vi "Add Sheets.vi"(8 "error in":errorcluster, 9 "Write/Read Cell":T1={"Cell Range"="", "Data 2D"=[], "Select Sheet"="", "1 Data"="", "Data 1D"=[], "Font col"=0, "Bold"=TRUE, "Font Size"=18, "Inside lines"=FALSE}, 10 "Work Sheet":refnum<k7>, 11 "Excel._Workbook":refnum<k7>) -> (0 "error out":errorcluster, 2 "Work Sheet":refnum<k7>, 3 "Excel._Workbook":refnum<k7>)   [LabVIEW 2017]
uses:
  controls/read.write.ctl
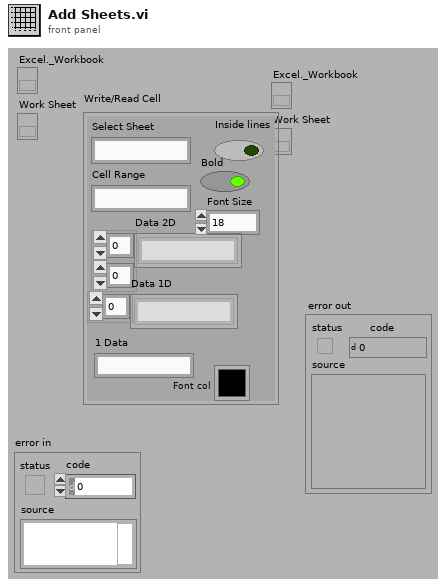
[diagram p1: front panel]
types:
  T1 = typedef "read.write.ctl" = cluster{"Cell Range":string, "Data 2D":string[][], "Select Sheet":string, "1 Data":string, "Data 1D":string[], "Font col":u32, "Bold":bool, "Font Size":i32, "Inside lines":bool}
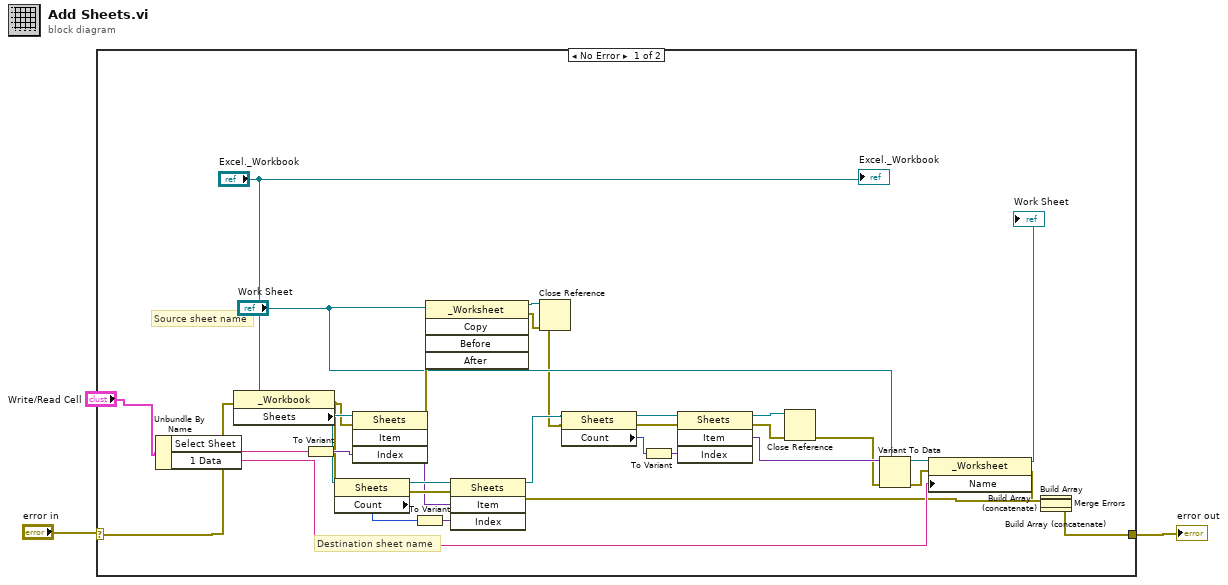
[diagram p0: block diagram]
diagram:
  n1 = case shown="No Error" "error in" {
    selector: "error in" -> [w30 w39]
    tunnel: [w7 w39] -> w1
    frame No Error {
      # "Source sheet name"
      # "Destination sheet name"
      n2 = Unbundle By Name("Write/Read Cell") -> ("Select Sheet"=w29:string, "1 Data"=w28:string)
      n3 = property class="_Workbook"(reference="Excel._Workbook", error in=w30) -> (error out=w15:errorcluster, "Sheets"=w16:refnum<k7>)  [unwired: 1 out]
      n4 = To Variant(anything=w29) -> (Variant=w32:variant)
      n5 = property class="Sheets"(reference=w16, error in=w15) -> (reference out=w17:refnum<k7>, error out=w18:errorcluster, "Count"=w13:i32)
      n6 = invoke class="Sheets" method="Item"(reference=w16, error in=w15, "Index"=w32) -> (error out=w25:errorcluster)  [unwired: 1 in, 3 out]
      n7 = To Variant(anything=w13) -> (Variant=w14:variant)
      n8 = invoke class="Sheets" method="Item"(reference=w17, error in=w18, "Index"=w14) -> (reference out=w11:refnum<k7>, error out=w9:errorcluster, "Item"=w12:variant)  [unwired: 1 in, 1 out]
      n9 = invoke class="_Worksheet" method="Copy"(reference="Work Sheet", error in=w25, "After"=w12) -> (reference out=w27:refnum<k7>, error out=w26:errorcluster)  [unwired: 2 in, 3 out]
      n10 = Close Reference(reference=w27, error in (no error)=w26) -> (error out=w10:errorcluster)
      n11 = property class="Sheets"(reference=w11, error in=w10) -> (reference out=w20:refnum<k7>, error out=w19:errorcluster, "Count"=w22:i32)
      n12 = To Variant(anything=w22) -> (Variant=w33:variant)
      n13 = invoke class="Sheets" method="Item"(reference=w20, error in=w19, "Index"=w33) -> (reference out=w34:refnum<k7>, error out=w38:errorcluster, "Item"=w35:variant)  [unwired: 1 in, 1 out]
      n14 = Close Reference(reference=w34, error in (no error)=w38) -> (error out=w24:errorcluster)
      n15 = Variant To Data(error in=w24, type="Work Sheet", Variant=w35) -> (data=w36:refnum<k7>, error out=w37:errorcluster)
      n16 = property class="_Worksheet"(reference=w36, error in=w37, "Name"=w28) -> (reference out=→"Work Sheet":refnum<k7>, error out=w8:errorcluster)
      n17 = Build Array(w8, w9) -> (w5:errorcluster[])
      n18 = Build Array (concatenate)(w5) -> (w4:errorcluster[])
      n19 = Build Array (concatenate)(w4) -> (w3:errorcluster[])
      n20 = Merge Errors(w3) -> (w7:errorcluster)
      "Excel._Workbook" <- "Excel._Workbook"
    }
    frame Error {
    }
  }
  "error out" <- w1
